vi "Read Comm to gRPC.vi"(8 "error in (no error)":errorcluster, 11 "CIFTemplatePlugin in":refnum<class "TemplatePlugin.lvclass">) -> (0 "error out":errorcluster, 3 "CIFTemplatePlugin out":refnum<class "TemplatePlugin.lvclass">)   [LabVIEW 2021, in "TemplatePlugin.lvclass"]
uses:
  TemplatePlugin.lvclass
  TemplatePlugin.lvclass/TemplatePlugin.ctl
  Common/Typedef/OOB Comm/To gRPC Command Payload.ctl
  Common/Typedef/OOB Comm/To gRPC Command.ctl
  Common/Typedef/OOB Comm/To gRPC Command Data.ctl
  <vilib>/CIF Foundation/CIF CIPC/TypeDefs/Read Configuration.ctl
  <vilib>/CIF Foundation/CIF CIPC/TypeDefs/Read Position.ctl
  f031ee7a-4e36-46a2-9ecb-acdc30148a67.vi
  4f85eb37-057c-4128-a96e-b37296c04816.vi
  <vilib>/CIF Foundation/CIF CIPC/SubVIs/Wait For N Elements Available.vi
  <vilib>/CIF Foundation/CIF CIPC/SubVIs/Check Error.vi
  <vilib>/CIF Foundation/CIF CIPC/SubVIs/Get dll Path.vi
  <vilib>/CIF Foundation/CIF CIPC/SubVIs/Get Element Read Position.vi
  <vilib>/CIF Foundation/CIF CIPC/SubVIs/Set Element Read Position.vi
  <vilib>/CIF Foundation/CIF CIPC/SubVIs/Get Element Info Variant.vi
  <vilib>/Utility/error.llb/Trim Whitespace.vi
  <vilib>/Utility/error.llb/Error Cluster From Error Code.vi
  <vilib>/CIF Foundation/CIF CIPC/CIF_NI_CIPC.lvlib
  Common/TemplateCommon.lvlib
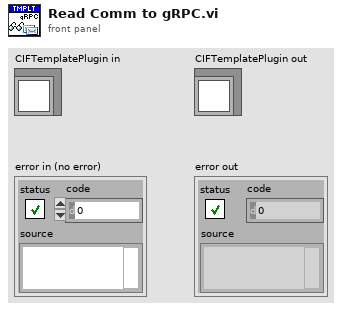
[diagram p1: front panel]
types:
  T1 = typedef "TemplateCommon.lvlib/To gRPC Command Payload.ctl" = cluster{"-> gRPC Command":T2, "-> gRPC Data":T3}
  T2 = typedef "TemplateCommon.lvlib/To gRPC Command.ctl" = enum16{"Read Data", "Read DVR Data"}
  T3 = typedef "TemplateCommon.lvlib/To gRPC Command Data.ctl" = cluster{"Cmd Data 1 -> gRPC":i32}
  T4 = typedef "Read Configuration.ctl" = cluster{"Read Position (Newest)":T5, "Element Offset":i32, "Prepend Array Size":bool, "Get Read Position":bool}
  T5 = typedef "CIF_NI_CIPC.lvlib/Read Position.ctl" = enum16{"Next", "Newest", "Oldest", "Next Available", "Absolute"}
  T6 = typedef "TemplateCommon.lvlib/To gRPC DVR Data.ctl" = cluster{"Data 1 DVR -> gRPC ":i32}
  T7 = typedef "TemplateCommon.lvlib/To gRPC Cyclic Data.ctl" = cluster{"Data 1 -> gRPC":i32}
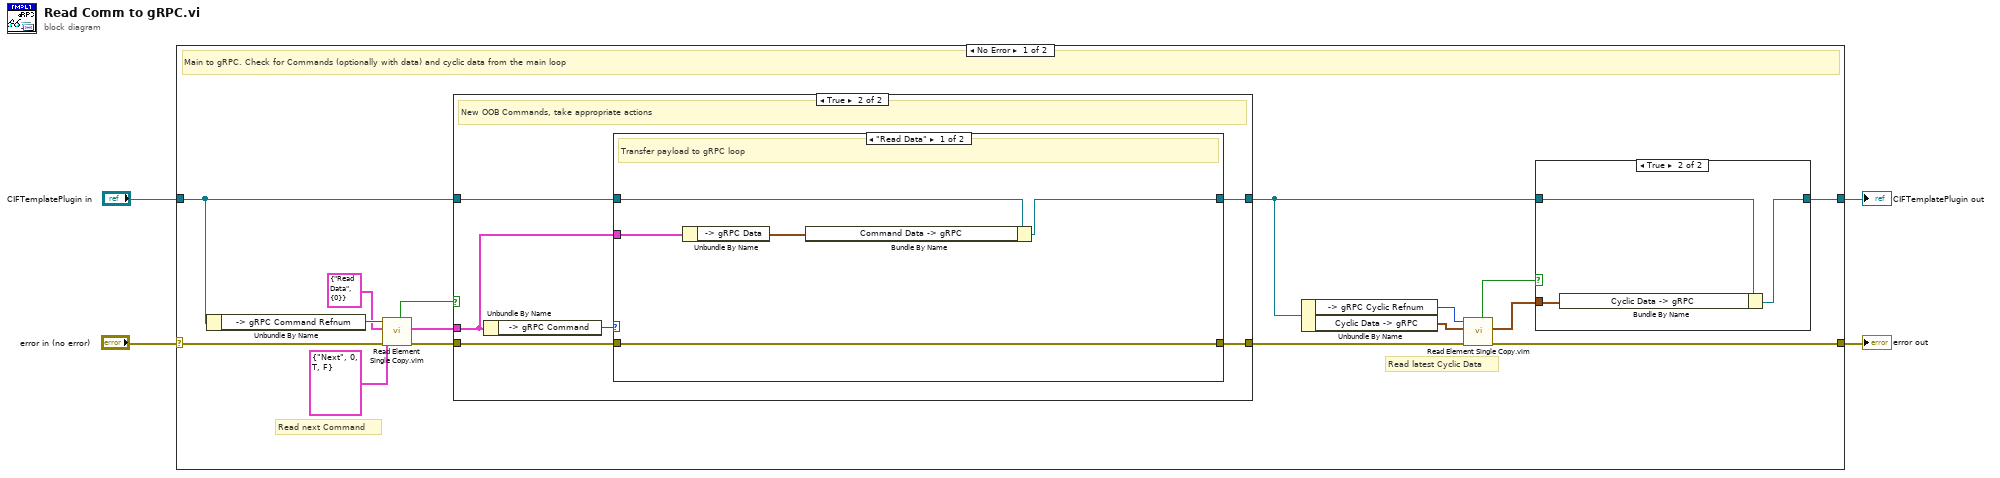
[diagram p0: block diagram]
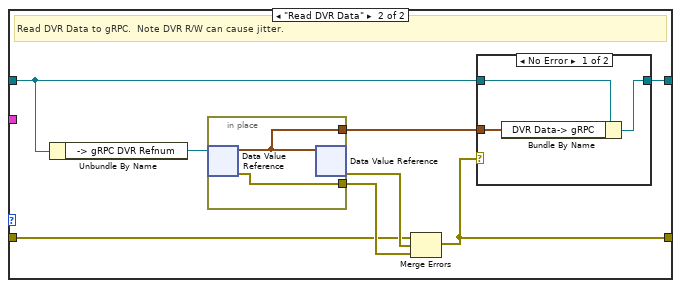
[diagram p4: hidden frame]
diagram:
  n1 = case shown="No Error" "error in (no error)" {
    selector: "error in (no error)" -> [w19 w53]
    tunnel: [w12 w53] -> w3
    tunnel: [w6 w52] -> w1
    tunnel: "CIFTemplatePlugin in" -> [w18 w52]
    frame No Error {
      # "Read next Command"
      # "Read latest Cyclic Data"
      # "Main to gRPC. Check for Commands (optionally with data) and cyclic data from the main loop"
      n2 = Unbundle By Name(w18) -> ("-> gRPC Command Refnum"=w20:u64)
      n3 = call "Read Element Single Copy.vim"("error in (no error)"=w19, "Read Configuration"=T4 {"Read Position (Newest)"=enum."Next", "Element Offset"=0, "Prepend Array Size"=TRUE, "Get Read Position"=FALSE}, "Data in"=T1 {"-> gRPC Command"=enum."Read Data", "-> gRPC Data"={"Cmd Data 1 -> gRPC"=0}} ("-> gRPC Payload"), "CIPC Reference in"=w20) -> ("error out"=w16:errorcluster, "Data out"=w15:T1, "Success"=w17:bool)  [unwired: 3 in, 2 out]
      n4 = case shown="True" w17 {
        tunnel: w18 -> [w26 w32]
        tunnel: [w26 w27] -> w7
        tunnel: w16 -> [w25 w31]
        tunnel: [w25 w30] -> w13
        tunnel: w15 -> [_ w28]
        frame False {
          # "No new OOB Commands"
        }
        frame True {
          # "New OOB Commands, take appropriate actions"
          n5 = Unbundle By Name(w28) -> ("-> gRPC Command"=w29:T2)
          n6 = case shown="\"Read Data\"" w29 {
            tunnel: w31 -> [w37 w41]
            tunnel: w32 -> [w35 w40]
            tunnel: [w37 w38] -> w30
            tunnel: w28 -> [w36 _]
            tunnel: [w33 w39] -> w27
            frame "Read Data" {
              # "Transfer payload to gRPC loop"
              n7 = Unbundle By Name(w36) -> ("-> gRPC Data"=w34:T3)
              n8 = Bundle By Name(cluster=w35, "Command Data -> gRPC"=w34) -> (w33:refnum<class "TemplatePlugin.lvclass">)
            }
            frame "Read DVR Data" {
              # "Read DVR Data to gRPC.  Note DVR R/W can cause jitter."
              n9 = Unbundle By Name(w40) -> ("-> gRPC DVR Refnum"=w43:refnum<data-value>)
              n10 = in-place {
                in-place-border: [w51] -> w45
                in-place-border: [w50] -> w42
                n11 = in-place-dvr #1(w43) -> (w50:T6, w51:errorcluster)
                n12 = in-place-dvr #1(w50) -> (w44:errorcluster)  [unwired: 1 out]
              }
              n13 = Merge Errors(w41, w44, w45) -> (w38:errorcluster)
              n14 = case shown="No Error" w38 {
                tunnel: w42 -> [w48 _]
                tunnel: w40 -> [w47 w49]
                tunnel: [w46 w49] -> w39
                frame No Error {
                  n15 = Bundle By Name(cluster=w47, "DVR Data-> gRPC"=w48) -> (w46:refnum<class "TemplatePlugin.lvclass">)
                }
                frame Error {
                }
              }
            }
          }
        }
      }
      n16 = Unbundle By Name(w7) -> ("-> gRPC Cyclic Refnum"=w14:u64, "Cyclic Data -> gRPC"=w11:T7)
      n17 = call "Read Element Single Copy.vim"("error in (no error)"=w13, "Data in"=w11, "CIPC Reference in"=w14) -> ("error out"=w12:errorcluster, "Data out"=w8:T7, "Success"=w9:bool)  [unwired: 4 in, 2 out]
      n18 = case shown="True" w9 {
        tunnel: w8 -> [_ w23]
        tunnel: w7 -> [w21 w24]
        tunnel: [w21 w22] -> w6
        frame False {
        }
        frame True {
          n19 = Bundle By Name(cluster=w24, "Cyclic Data -> gRPC"=w23) -> (w22:refnum<class "TemplatePlugin.lvclass">)
        }
      }
    }
    frame Error {
    }
  }
  "error out" <- w3
  "CIFTemplatePlugin out" <- w1
